vi "Analog_AI_AO.vi"() -> (4 "Timeout (s)":dbl, 6 "Input task":refnum<k21>, 8 "AO Output task":refnum<k21>, 10 "error out":errorcluster, 15 "Array of Piezo and Pockels Task":refnum<k21>[](array[refnum]))   [LabVIEW 2017]
uses:
  Custom Controls/scan mode main settings tab.ctl
  Custom Controls/advanced settings inner tab CTL.ctl
  <vilib>/DAQmx/write.llb/DAQmx Write (Analog 1D Wfm NChan NSamp).vi
  GFG/GFGnumericGet.vi
  GFG/GFGbooleanGet.vi
  GFG/GFGstringGet.vi
  <vilib>/Waveform/WDTOps.llb/WDT Number of Waveform Samples DBL.vi
  <vilib>/DAQmx/configure/timing.llb/DAQmx Timing (Sample Clock).vi
  <vilib>/DAQmx/configure/trigger.llb/DAQmx Start Trigger (Digital Edge).vi
  <vilib>/DAQmx/create/channels.llb/DAQmx Create Channel (AO-Voltage-Basic).vi
  <vilib>/DAQmx/configure/timing.llb/DAQmx Timing (Use Waveform).vi
  <vilib>/DAQmx/miscellaneous.llb/DAQmx Fill In Error Info.vi
  GFG/GFG library.lvlib
  <resource>/objmgr/daqmx.rc
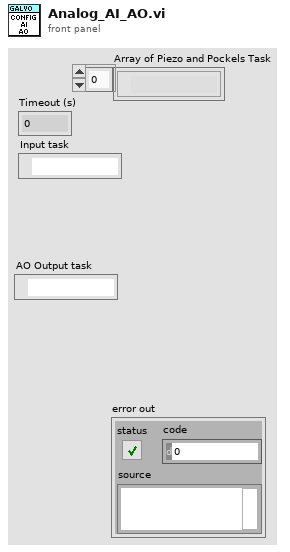
[diagram p1: front panel]
types:
  T1 = typedef "scan mode main settings tab.ctl" = enum32{"2D frame", "2D line scan", "general settings", "Z Stack", "piezo"}
  T2 = typedef "advanced settings inner tab CTL.ctl" = enum32{"arb. frames", "AO", "AI", "channels", "trigger", "Zstack data"}
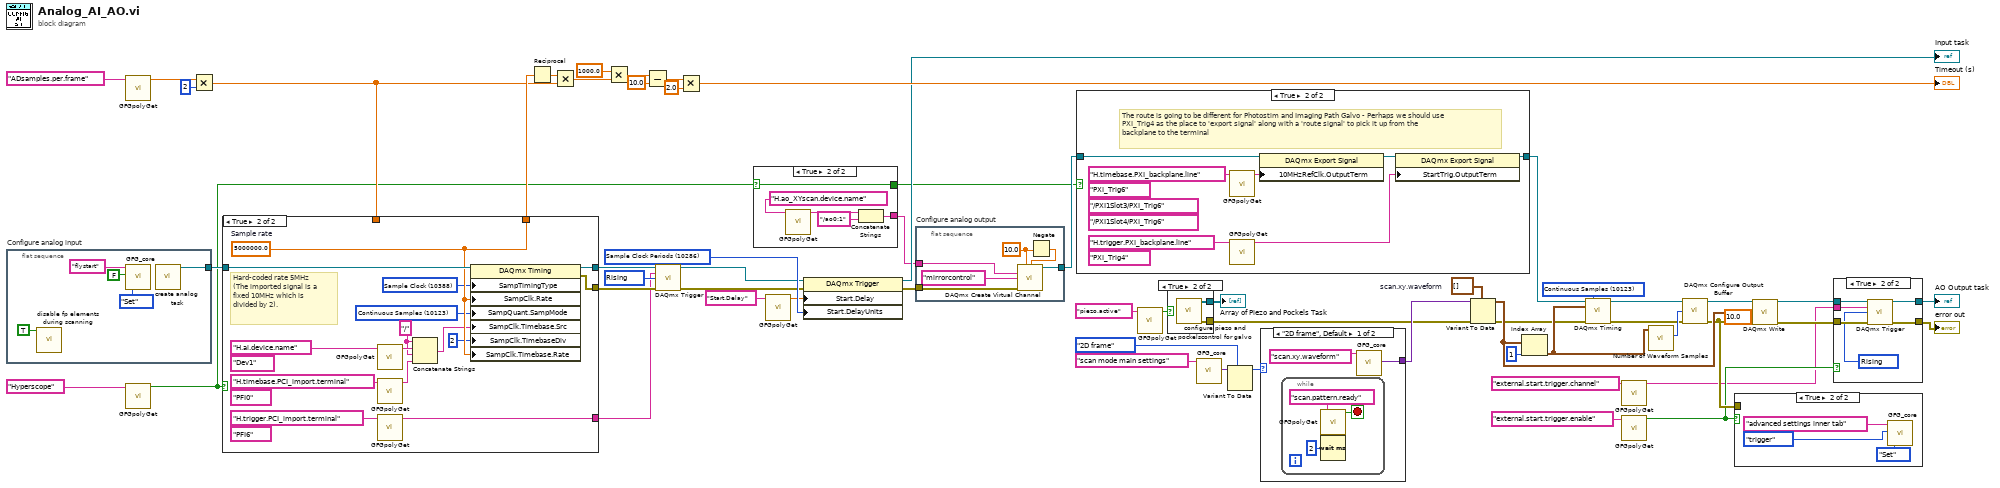
[diagram p0: block diagram]
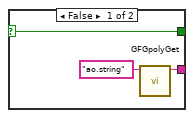
[diagram p2: hidden frame]
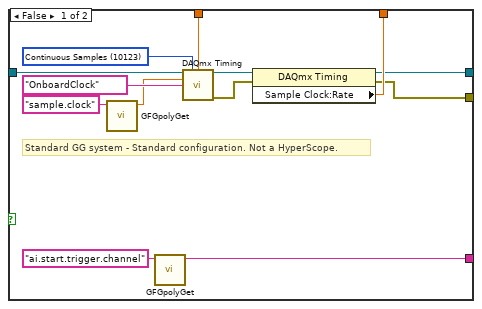
[diagram p4: hidden frame]
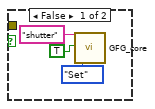
[diagram p6: hidden frame]
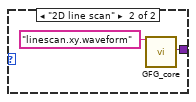
[diagram p8: hidden frame]
diagram:
  w12 = 10280 items=["Rising"=10280, "Falling"=10171] ("Slope")
  w19 = 10286 items=["Sample Clock Periods"=10286, "Seconds"=10364, "Ticks"=10304] ("Start.DelayUnits")
  w30 = 10123 items=["Finite Samples"=10178, "Continuous Samples"=10123] ("sample mode")
  w41 = waveform(dbl)[] []  # scan.xy.waveform
  n1 = flat-sequence "Configure analog input" {
    tunnel: [w65] -> w60
    frame #0 {
      n2 = call "disable fp elements during scanning.vi"("T for grey out"=TRUE) -> ()  [unwired: 11 in]
      n3 = call "GFG_core.vi"("Variable Name in"="flystart", "Variant in"=FALSE ("NewVal"), "Action"=enum16{"Init", "Set", "Get"}."Set") -> ()  [unwired: 10 in, 7 out]
      n4 = call "create analog task.vi"() -> ("task out"=w65:refnum<k21>)  [unwired: 11 in]
    }
  }
  n5 = call-poly "GFGpolyGet.vi"("Variable Name in"="ADsamples.per.frame" ("Tag in")) -> ("Numeric"=w53:dbl)  [unwired: 8 in, 2 out]
  n6 = call-poly "GFGpolyGet.vi"("Variable Name in"="Hyperscope") -> ("Boolean Value OUT"=w3:bool)  [unwired: 9 in, 1 out]
  n7 = Multiply(x=w53, y=i8 2) -> (x*y=w52:dbl)
  n8 = case shown="True" w3 {
    tunnel: w60 -> [w78 w93]
    tunnel: [w72 w92] -> w57
    tunnel: w52 -> [w71 _]
    tunnel: [w69 w91] -> w14
    tunnel: [w70 w90] -> w13
    tunnel: [w66 w88] -> w9
    frame False {
      w68 = 10123 items=["Finite Samples"=10178, "Continuous Samples"=10123] ("sample mode")
      # "Standard GG system - Standard configuration. Not a HyperScope."
      n9 = call-poly "GFGpolyGet.vi"("Variable Name in"="sample.clock" ("Tag in")) -> ("Numeric"=w75:dbl)  [unwired: 8 in, 2 out]
      n10 = call-poly "GFGpolyGet.vi"("Variable Name in"="ai.start.trigger.channel" ("Tag in")) -> ("String"=w66:string)  [unwired: 9 in, 1 out]
      n11 = call-poly <vilib>:"DAQmx Timing.vi"("task/channels in"=w78, "sample mode"=w68, "samples per channel"=w71, "rate"=w75, "source"=tag "OnboardClock") -> ("task out"=w74:refnum<k21>, "error out"=w73:errorcluster)  [unwired: 9 in]
      n12 = property class="DAQmx Timing"(reference=w74, error in=w73) -> (reference out=w70:refnum<k21>, error out=w69:errorcluster, "Sample Clock:Rate"=w72:dbl)
    }
    frame True {
      (unwired) tag "Dev1" ("Output Terminal")
      w80 = "/" ("string")
      (unwired) tag "PFI0" ("Output Terminal")
      w92 = 5000000.0  # Sample rate
      w86 = 10388 items=["Sample Clock"=10388, "Burst Handshake"=12548, "Handshake"=10389, "Implicit"=10451, "On Demand"=10390, "Change Detection"=12504, "Pipelined Sample Clock"=14668] ("SampTimingType")
      w87 = 10123 items=["Finite Samples"=10178, "Continuous Samples"=10123, "Hardware Timed Single Point"=12522] ("SampQuant.SampMode")
      (unwired) tag "PFI6" ("Output Terminal")
      # "Hard-coded rate 5MHz\n(The imported signal is a fixed 10MHz which is divided by 2)."
      n13 = call-poly "GFGpolyGet.vi"("Variable Name in"="H.ai.device.name" ("Tag in")) -> ("String"=w81:string)  [unwired: 9 in, 1 out]
      n14 = call-poly "GFGpolyGet.vi"("Variable Name in"="H.timebase.PCI_import.terminal" ("Tag in")) -> ("String"=w82:string)  [unwired: 9 in, 1 out]
      n15 = call-poly "GFGpolyGet.vi"("Variable Name in"="H.trigger.PCI_import.terminal" ("Tag in")) -> ("String"=w88:string)  [unwired: 9 in, 1 out]
      n16 = Concatenate Strings(w80, w81, w80, w82) -> (w79:string)
      n17 = property class="DAQmx Timing"(reference=w93, "SampTimingType"=w86, "SampClk.Rate"=w92, "SampQuant.SampMode"=w87, "SampClk.Timebase.Src"=w79, "SampClk.TimebaseDiv"=u32 2, "SampClk.Timebase.Rate"=w92) -> (reference out=w90:refnum<k21>, error out=w91:errorcluster)  [unwired: 1 in]
    }
  }
  n18 = Reciprocal(x=w57) -> (1/x=w56:dbl)
  n19 = Multiply(x=w56, y=w52) -> (x*y=w55:dbl)
  n20 = Multiply(x=1000.0, y=w55) -> (x*y=w48:dbl)
  n21 = Subtract(x=w48, y=10.0) -> (x-y=w51:dbl)
  n22 = call-poly <vilib>:"DAQmx Trigger.vi"("task/channels in"=w13, "source"=w9, "edge"=w12, "error in"=w14) -> ("task out"=w10:refnum<k21>, "error out"=w11:errorcluster)  [unwired: 10 in]
  n23 = Multiply(x=w51, y=2.0) -> (x*y=→"Timeout (s)":dbl)
  n24 = case shown="True" w3 {
    selector: w3 -> [w96 w101]
    tunnel: [w96 w101] -> w2
    tunnel: [w94 w97] -> w1
    frame False {
      n25 = call-poly "GFGpolyGet.vi"("Variable Name in"="ao.string" ("name to assign")) -> ("String"=w94:string)  [unwired: 9 in, 1 out]
    }
    frame True {
      n26 = call-poly "GFGpolyGet.vi"("Variable Name in"="H.ao_XYscan.device.name" ("name to assign")) -> ("String"=w99:string)  [unwired: 9 in, 1 out]
      n27 = Concatenate Strings(w99, "/ao0:1" ("string")) -> (w97:string)
    }
  }
  n28 = call-poly "GFGpolyGet.vi"("Variable Name in"="Start.Delay" ("Tag in")) -> ("Numeric"=w18:dbl)  [unwired: 8 in, 2 out]
  n29 = property class="DAQmx Trigger"(reference=w10, error in=w11, "Start.Delay"=w18, "Start.DelayUnits"=w19) -> (reference out=→"Input task":refnum<k21>, error out=w15:errorcluster)
  n30 = flat-sequence "Configure analog output" {
    tunnel: [w106] -> w6
    tunnel: w15 -> [w103]
    tunnel: w1 -> [w102]
    frame #0 {
      w104 = 10.0 ("maximum value")
      n31 = Negate(x=w104) -> (-x=w105:dbl)
      n32 = call-poly <vilib>:"DAQmx Create Virtual Channel.vi"("maximum value"=w104, "minimum value"=w105, "physical channels"=w102, "name to assign"="mirrorcontrol", "error in"=w103) -> ("task out"=w106:refnum<k21>)  [unwired: 9 in, 1 out]
    }
  }
  n33 = case shown="True" w2 {
    tunnel: [w108 w114] -> w7
    tunnel: w6 -> [w108 w113]
    frame False {
      # "NOT A HYPERSCOPE!"
    }
    frame True {
      (unwired) tag "PXI_Trig6" ("Output Terminal")
      (unwired) tag "/PXI1Slot4/PXI_Trig6" ("Output Terminal")
      (unwired) tag "/PXI1Slot3/PXI_Trig6" ("Output Terminal")
      (unwired) tag "PXI_Trig4" ("StartTrig.OutputTerm")
      # "The route is going to be different for Photostim and Imaging Path Galvo - Perhaps we should use PXI_Trig4 as the place to 'export signal' along with a 'route signal' to pick it up from the backplane to the terminal"
      n34 = call-poly "GFGpolyGet.vi"("Variable Name in"="H.timebase.PXI_backplane.line") -> ("String"=w109:string)  [unwired: 9 in, 1 out]
      n35 = call-poly "GFGpolyGet.vi"("Variable Name in"="H.trigger.PXI_backplane.line") -> ("String"=w111:string)  [unwired: 9 in, 1 out]
      n36 = property class="DAQmx Export Signal"(reference=w113, "10MHzRefClk.OutputTerm"=w109) -> (reference out=w115:refnum<k21>)  [unwired: 1 in, 1 out]
      n37 = property class="DAQmx Export Signal"(reference=w115, "StartTrig.OutputTerm"=w111) -> (reference out=w114:refnum<k21>)  [unwired: 1 in, 1 out]
    }
  }
  n38 = call-poly "GFGpolyGet.vi"("Variable Name in"="piezo.active") -> ("Boolean Value OUT"=w25:bool)  [unwired: 9 in, 1 out]
  n39 = case shown="True" w25 {
    tunnel: [_ w117] -> w24
    tunnel: [_ w116] -> w8
    frame False {
    }
    frame True {
      n40 = call "configure piezo and pockelscontrol for galvo.vi"() -> ("error out"=w117:errorcluster, "Array of Piezo and Pockels Task"=w116:refnum<k21>[])  [unwired: 10 in]
    }
  }
  "Array of Piezo and Pockels Task" <- w8
  n41 = call "GFG_core.vi"("Variable Name in"="scan mode main settings") -> ("Variant Out"=w37:variant)  [unwired: 12 in, 6 out]
  n42 = Variant To Data(type=scan_mode_main_settings_tab."2D frame" ("scan mode main settings"), Variant=w37) -> (data=w35:T1)  [unwired: 1 in, 1 out]
  n43 = case shown="\"2D frame\", Default" w35 {
    tunnel: [w118 w123] -> w40
    frame "2D frame", Default {
      n44 = while {
        stop <- w121 stop-if-true
        n45 = call-poly "GFGpolyGet.vi"("Variable Name in"="scan.pattern.ready") -> ("Boolean Value OUT"=w121:bool)  [unwired: 9 in, 1 out]
        n46 = Wait (ms)(milliseconds to wait=u32 2) -> ()  [unwired: 1 out]
      }
      n47 = call "GFG_core.vi"("Variable Name in"="scan.xy.waveform") -> ("Variant Out"=w118:variant)  [unwired: 12 in, 6 out]
    }
    frame "2D line scan" {
      n48 = call "GFG_core.vi"("Variable Name in"="linescan.xy.waveform") -> ("Variant Out"=w123:variant)  [unwired: 12 in, 6 out]
    }
  }
  n49 = Variant To Data(error in=w24, type=w41, Variant=w40) -> (data=w39:waveform(dbl)[], error out=w29:errorcluster)
  n50 = Index Array(array=w39, index=1) -> (element=w44:waveform(dbl))
  n51 = call-poly <vilib>:"DAQmx Timing.vi"("task/channels in"=w7, "sample mode"=w30, "waveform"=w44, "error in"=w29) -> ("task out"=w42:refnum<k21>, "error out"=w38:errorcluster)  [unwired: 10 in]
  n52 = call-poly "GFGpolyGet.vi"("Variable Name in"="external.start.trigger.channel" ("Tag in")) -> ("String"=w4:string)  [unwired: 9 in, 1 out]
  n53 = call-poly "GFGpolyGet.vi"("Variable Name in"="external.start.trigger.enable" ("Tag in")) -> ("Boolean Value OUT"=w27:bool)  [unwired: 9 in, 1 out]
  n54 = call-poly <vilib>:"Number of Waveform Samples.vi"("waveform in"=w44) -> ("number of samples"=w45:i32)  [unwired: 8 in, 2 out]
  n55 = call <vilib>:"DAQmx Configure Output Buffer.vi"("task/channels in"=w42, "buffer size (in samples per channel)"=w45, "error in"=w38) -> ("task out"=w46:refnum<k21>, "error out"=w31:errorcluster)  [unwired: 11 in]
  n56 = case shown="True" w27 {
    tunnel: w31 -> [_ _]
    frame False {
      n57 = call "GFG_core.vi"("Variable Name in"="shutter" ("Tag in"), "Variant in"=TRUE, "Action"=enum16{"Init", "Set", "Get"}."Set") -> ()  [unwired: 10 in, 7 out]
    }
    frame True {
      n58 = call "GFG_core.vi"("Variable Name in"="advanced settings inner tab", "Variant in"=advanced_settings_inner_tab_CTL."trigger" ("advanced settings inner tab"), "Action"=enum16{"Init", "Set", "Get", "Clear"}."Set") -> ()  [unwired: 10 in, 7 out]
    }
  }
  n59 = call-poly <vilib>:"DAQmx Write.vi"("task/channels in"=w46, "data"=w39, "timeout"=10.0 ("Wirite Timeout"), "error in"=w31) -> ("task out"=w33:refnum<k21>, "error out"=w28:errorcluster)  [unwired: 9 in, 1 out]
  n60 = case shown="True" w27 {
    tunnel: w4 -> [_ w138]
    tunnel: w33 -> [w132 w137]
    tunnel: [w132 w136] -> w22
    tunnel: w28 -> [w131 w135]
    tunnel: [w131 w134] -> w21
    frame False {
    }
    frame True {
      w133 = 10280 items=["Rising"=10280, "Falling"=10171] ("edge")
      n61 = call-poly <vilib>:"DAQmx Trigger.vi"("task/channels in"=w137, "source"=w138, "edge"=w133, "error in"=w135) -> ("task out"=w136:refnum<k21>, "error out"=w134:errorcluster)  [unwired: 10 in]
    }
  }
  "AO Output task" <- w22
  "error out" <- w21
